vi "Set DAQ Offset.vi"(8 "error in (no error)":errorcluster, 10 "Offsets":dbl[](array[numeric]), 11 "Instrument.DAQ":refnum<class "Instrument.DAQ.lvclass">) -> (0 "error out":errorcluster, 3 "Instrument.DAQ out":refnum<class "Instrument.DAQ.lvclass">)   [LabVIEW 2019, in "Instrument.Lockin.lvlib" / "Instrument.DAQ.lvclass"]
uses:
  Instrument.DAQ.lvclass
  Instrument.DAQ.lvclass/Instrument.DAQ.ctl
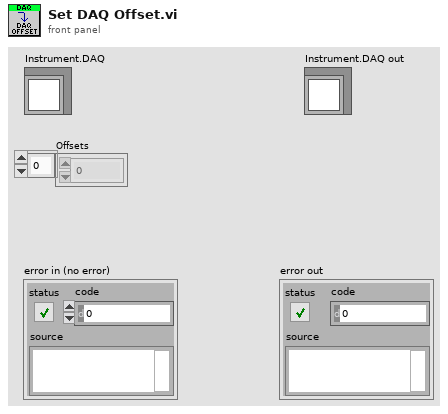
[diagram p1: front panel]
types:
  T1 = typedef "Instrument.Lockin.lvlib/Instrument.DAQ.lvclass/Channel.Gain--Cluster--Array.ctl" = T2[]
  T2 = typedef "Instrument.Lockin.lvlib/Instrument.DAQ.lvclass/Channel.Gain--Cluster.ctl" = cluster{"Channel":string, "Gain":dbl}
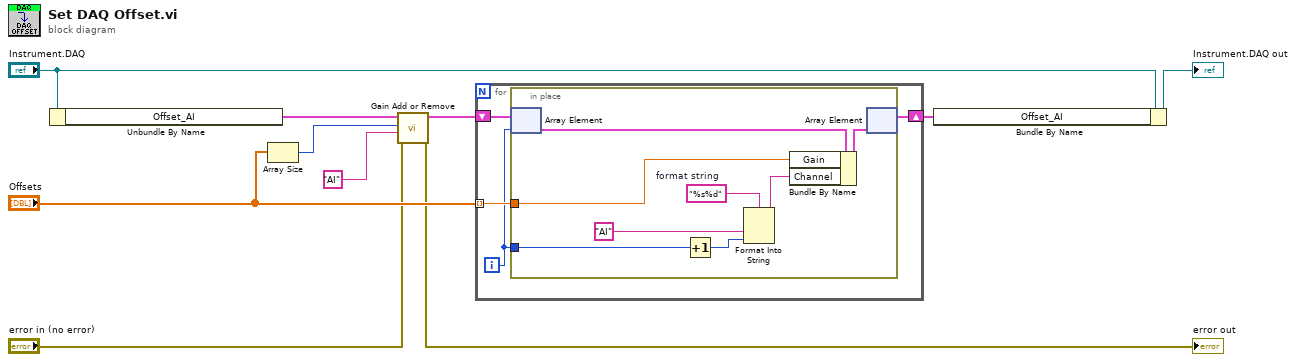
[diagram p0: block diagram]
diagram:
  n1 = Unbundle By Name("Instrument.DAQ") -> ("Offset_AI"=w2:T1)
  n2 = Array Size(array="Offsets") -> (size(s)=w7:i32)
  n3 = call "Gain Add or Remove.vi"("error in (no error)"="error in (no error)", "Name Prefix"="AI", "Size"=w7, "Channel Gain"=w2) -> ("error out"=→"error out":errorcluster, "Channel Gain out"=w5:T1)  [unwired: 6 in]
  n4 = for {
    tunnel: "Offsets" -> [w14] mode=indexing
    shift-right: [w11] -> w8
    shift-left: w5 -> [w13]
    i -> [w12]
    n5 = in-place {
      in-place-border: w12 -> [w22]
      in-place-border: w14 -> [w18]
      w21 = "%s%d"  # format string
      n6 = in-place-array #1(w13, w12) -> (w15:T2)
      n7 = Increment(x=w22) -> (x+1=w19:i32)
      n8 = Format Into String(format string=w21, "AI" ("input 1"), w19) -> (resulting string=w20:string)  [unwired: 2 in, 1 out]
      n9 = Bundle By Name(cluster=w15, "Gain"=w18, "Channel"=w20) -> (w16:T2)
      n10 = in-place-array #1(w16) -> (w11:T1)  [unwired: 1 out]
    }
  }
  n11 = Bundle By Name(cluster="Instrument.DAQ", "Offset_AI"=w8) -> (→"Instrument.DAQ out":refnum<class "Instrument.DAQ.lvclass">)
